vi "dvp Vi Get Noise Reduct3d State.vi"(10 "pNoiseReduct3dState":i32, 11 "handle":u32) -> (2 "pNoiseReduct3dState out":i32, 3 "function return":u32(ring))   [LabVIEW 2018, in "LabViewDVPCamera.lvlib"]
doc: "LabviewDvp2Api dvpStatus dvpViGetNoiseReduct3dState(dvpHandle handle, BOOL *pNoiseReduct3dState);"
uses:
  LabViewDVPCamera.lvlib
  LabViewDVPCamera/LabViewDVPCamera.dll
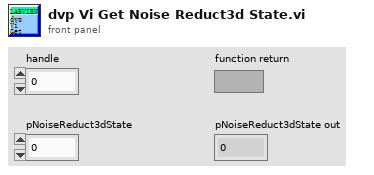
[diagram p1: front panel]
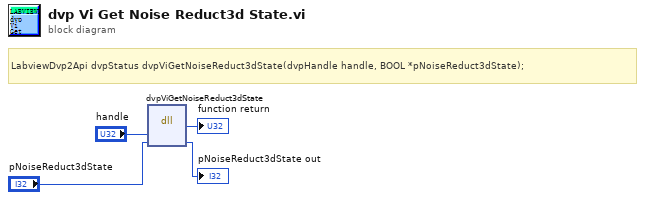
[diagram p0: block diagram]
diagram:
  # "LabviewDvp2Api dvpStatus dvpViGetNoiseReduct3dState(dvpHandle handle, BOOL *pNoiseReduct3dState);"
  n1 = dll-call lib="C:/Program Files (x86)/DVP2 Labview cn 64/Sample/LabViewDVPCamera/LabViewDVPCamera.*" fn="dvpViGetNoiseReduct3dState"("handle"="handle", "pNoiseReduct3dState"="pNoiseReduct3dState") -> (→"function return":u32, "pNoiseReduct3dState"=→"pNoiseReduct3dState out":i32)  [unwired: 4 in, 2 out]
